vi "Display.vi"(0 "reference in":refnum<class "CurrentConditionDisplay.lvclass">, 5 "error in (no error)":errorcluster) -> (14 "reference out":refnum<class "CurrentConditionDisplay.lvclass">, 16 "WeatherData":T1, 19 "error out":errorcluster)   [LabVIEW 2010, in "CurrentConditionDisplay.lvclass"]
uses:
  CurrentConditionDisplay.lvclass
  WeatherData.ctl
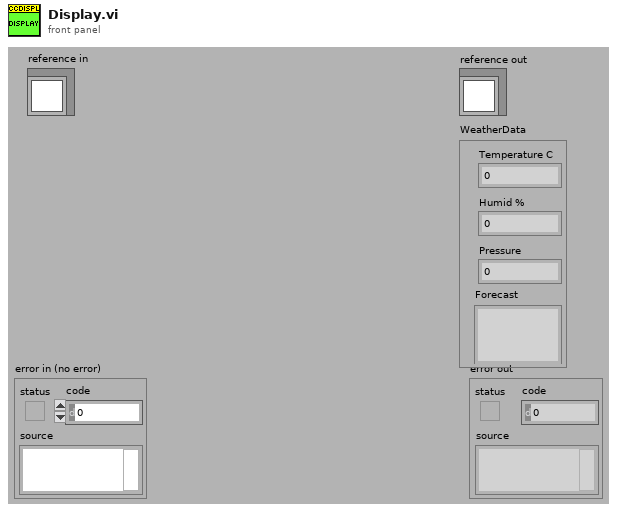
[diagram p1: front panel]
types:
  T1 = typedef "WeatherData.ctl" = cluster{"Temperature C":dbl, "Humid %":dbl, "Pressure":dbl, "Forecast":string}
  T2 = typedef "CurrentConditionDisplay.lvclass/ObjectAttributes.ctl" = cluster{"WeatherData":T1}
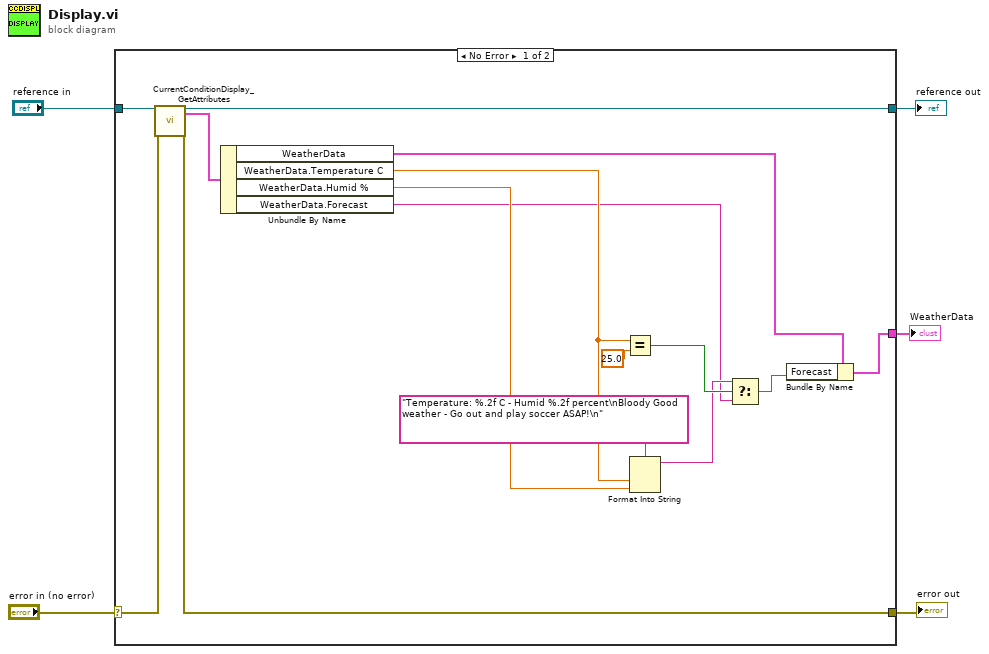
[diagram p0: block diagram]
diagram:
  n1 = case shown="No Error" "error in (no error)" {
    selector: "error in (no error)" -> [w20 w22]
    tunnel: [w18 w22] -> w4
    tunnel: [w16 w21] -> w2
    tunnel: "reference in" -> [w17 w21]
    tunnel: [w12 _] -> w1
    frame No Error {
      n2 = call "CurrentConditionDisplay_GetAttributes.vi"("reference in"=w17, "error in (no error)"=w20) -> ("reference out"=w16:refnum<class "CurrentConditionDisplay.lvclass">, "Data"=w19:T2, "error out"=w18:errorcluster)  [unwired: 14 in, 1 out]
      n3 = Unbundle By Name(w19) -> ("WeatherData"=w13:T1, "WeatherData.Temperature C"=w11:dbl, "WeatherData.Humid %"=w14:dbl, "WeatherData.Forecast"=w7:string)
      n4 = Equal?(x=w11, y=25.0) -> (x = y?=w9:bool)
      n5 = Format Into String(format string="Temperature: %.2f C - Humid %.2f percent\nBloody Good weather - Go out and play soccer ASAP!\n", w11, w14) -> (resulting string=w8:string)  [unwired: 2 in, 1 out]
      n6 = Select(t=w8, s=w9, f=w7) -> (s? t:f=w6:string)
      n7 = Bundle By Name(cluster=w13, "Forecast"=w6) -> (w12:T1)
    }
    frame Error {
    }
  }
  "error out" <- w4
  "reference out" <- w2
  "WeatherData" <- w1
